vi "box catch calculate.vi"(11 "main.ctl":T1) -> (0 "register address":i32, 1 "box position":cluster{i32, i32}, 3 "output cluster":T1)   [LabVIEW 2019]
uses:
  main data.ctl
  vision/vision_board_ctl.ctl
  block box.ctl
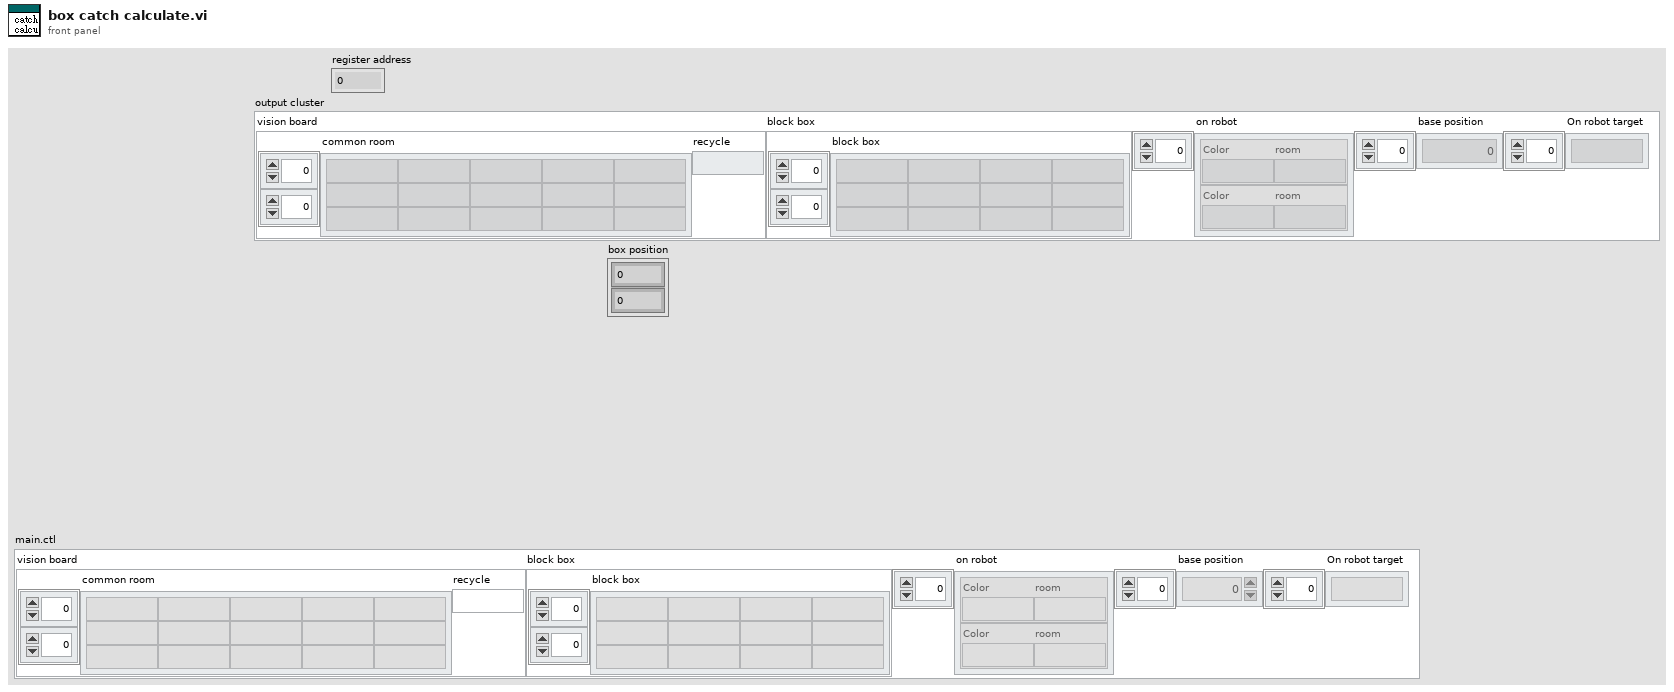
[diagram p1: front panel]
types:
  T1 = typedef "main data.ctl" = cluster{"vision board":T2, "block box":T3, "on robot ":cluster{"Color":string, "room":string}[], "base position":dbl[], "On robot target":string[]}
  T2 = typedef "vision_board_ctl.ctl" = cluster{"common room":string[][], "recycle":string}
  T3 = typedef "block box.ctl" = cluster{"block box":string[][]}
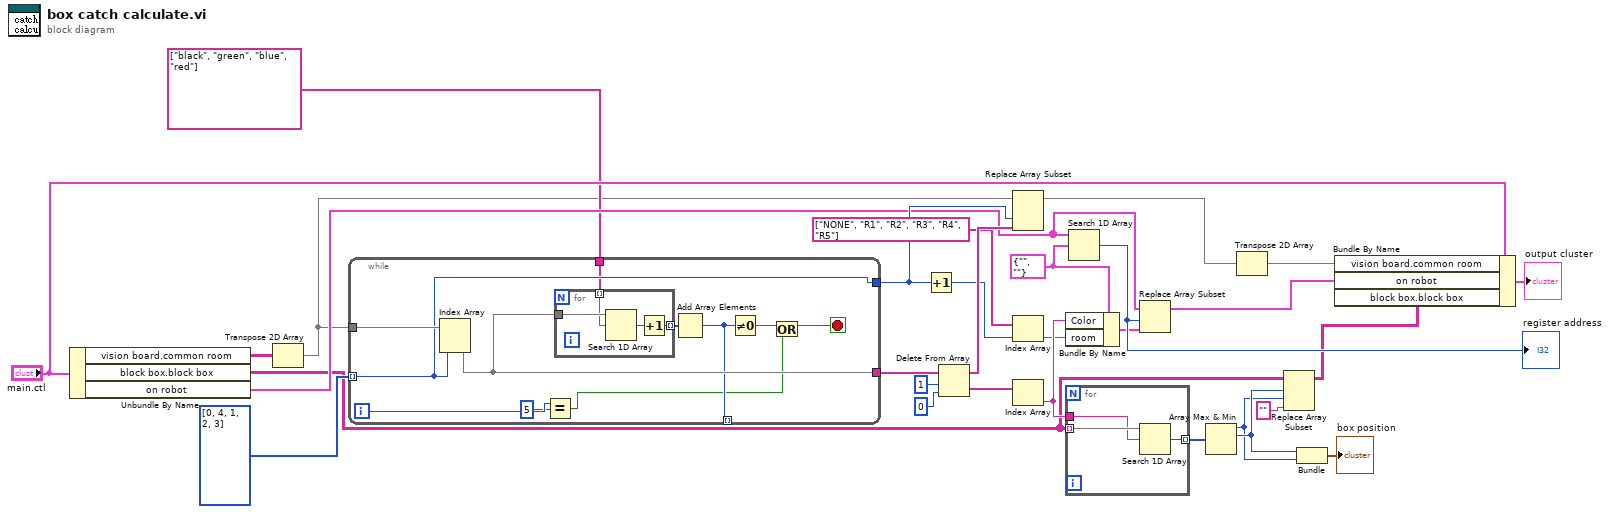
[diagram p0: block diagram]
diagram:
  w19 = cluster{"Color":string, "room":string} {"Color"="", "room"=""} ("Cluster")
  n1 = Unbundle By Name("main.ctl") -> ("vision board.common room"=w25:string[][], "block box.block box"=w10:string[][], "on robot"=w16:cluster{"Color":string, "room":string}[])
  n2 = Transpose 2D Array(2D array=w25) -> (transposed array=w2:string[][])
  n3 = while {
    tunnel: w2 -> [w41]
    tunnel: i32[] [0, 4, 1, 2, 3] -> [w38] mode=indexing
    tunnel: [w40] -> w29
    tunnel: [w38] -> w22
    tunnel: [w35] -> _ mode=indexing
    tunnel: string[] ["black", "green", "blue", "red"] -> [w36]
    i -> [w34]
    stop <- w32 stop-if-true
    n4 = Index Array(array=w41, index (col)=w38) -> (element=w40:string[])  [unwired: 1 in]
    n5 = Equal?(x=w34, y=5) -> (x = y?=w31:bool)
    n6 = for {
      tunnel: w40 -> [w45]
      tunnel: [w42] -> w37 mode=indexing
      tunnel: w36 -> [w43] mode=indexing
      n7 = Search 1D Array(1D array=w45, element=w43) -> (index of element=w44:i32)  [unwired: 1 in]
      n8 = Increment(x=w44) -> (x+1=w42:i32)
    }
    n9 = Add Array Elements(numeric array=w37) -> (sum=w35:i32)
    n10 = Not Equal To 0?(x=w35) -> (x != 0?=w39:bool)
    n11 = Or(x=w39, y=w31) -> (x .or. y?=w32:bool)
  }
  n12 = Increment(x=w22) -> (x+1=w21:i32)
  n13 = Delete From Array(array=w29, length=1, index=0) -> (deleted portion=w26:string[], array with subset deleted=w24:string[])
  n14 = Replace Array Subset(array=w2, new element=w24, index (col)=w22) -> (w12:string[][])  [unwired: 1 in]
  n15 = Index Array(array=string[] ["NONE", "R1", "R2", "R3", "R4", "R5"], index=w21) -> (element=w17:string)
  n16 = Index Array(array=w26) -> (element=w18:string)  [unwired: 1 in]
  n17 = Bundle By Name(cluster=w19, "Color"=w18, "room"=w17) -> (w14:cluster{"Color":string, "room":string})
  n18 = for {
    tunnel: w10 -> [w48] mode=indexing
    tunnel: w18 -> [w47]
    tunnel: [w46] -> w23 mode=indexing
    n19 = Search 1D Array(1D array=w48, element=w47) -> (index of element=w46:i32)  [unwired: 1 in]
  }
  n20 = Search 1D Array(1D array=w16, element=w19) -> (index of element=w15:i32)  [unwired: 1 in]
  "register address" <- w15
  n21 = Replace Array Subset(array=w16, new element=w14, index=w15) -> (w11:cluster{"Color":string, "room":string}[])
  n22 = Array Max & Min(array=w23) -> (max value=w5:i32, max index (indices)=w6:i32)  [unwired: 2 out]
  n23 = Transpose 2D Array(2D array=w12) -> (transposed array=w1:string[][])
  n24 = Replace Array Subset(array=w10, new element="" ("new element/subarray"), index (row)=w6, index (col)=w5) -> (w8:string[][])
  n25 = Bundle(w6, w5) -> (→"box position":cluster{i32, i32})  [unwired: 1 in]
  n26 = Bundle By Name(cluster="main.ctl", "vision board.common room"=w1, "on robot"=w11, "block box.block box"=w8) -> (→"output cluster":T1)
